vi "Inst.Transport.AppLauncher.vi"(8 "error in":errorcluster, 11 "Debug Mode":bool) -> (0 "error out":errorcluster)   [LabVIEW 2019, in "Inst.Transport.lvclass"]
uses:
  Inst.Transport.lvclass
  <vilib>/JKI/JKI SMO/SMO/Typedefs/SMOState --Enum.ctl
  <userlib>/LevyLab/Instrument Framework/Instrument/Instrument.lvclass
  <userlib>/LevyLab/Instrument Framework/Instrument UI/Instrument UI.lvclass
  C:/Program Files (x86)/National Instruments/LabVIEW 2019/vi.lib/JKI/JKI SMO/SMO/SMO.lvclass
  C:/Program Files (x86)/National Instruments/LabVIEW 2019/vi.lib/JKI/JKI SMO/SMO.UI/SMO.UI.lvclass
  C:/Program Files (x86)/National Instruments/LabVIEW 2019/user.lib/LevyLab/Instrument Framework/Instrument/Instrument.lvclass
  <vilib>/JKI/JKI SMO/SMO/SMO.lvclass/SMO.ctl
  <vilib>/JKI/JKI SMO/SMO/Private/ReftoDVR--SMO.vi
  <vilib>/JKI/JKI SMO/SMO/SMO.lvclass
  <vilib>/JKI/JKI SMO/SMO.UI/SMO.UI.lvclass
panel:
  in  "UI":bool
  in  "Examine Configuration.ini":bool
  in  "Splash Status":string="Push Start to Start..." caption="String"
  in  "Start Application":bool caption="Play"
  in  "Stop Application":bool caption="Stop"
  out "UI SMO State":T1=enum."Stopped"
  out "SMO State":T1
  # "Example Instrument SMO Test Launcher"
  # "For instructions on how to use the JKI State Machine Objects, examples and video tutorials, visit:\nhttp://jki.net/state-machine-objects/\n\nJKI State Machine Objects™\nhttp://jki.net/state-machine-objects/\nCopyright (C) 2005-2015, JKI <info@jki.net>\nALL RIGHTS RESERVED"
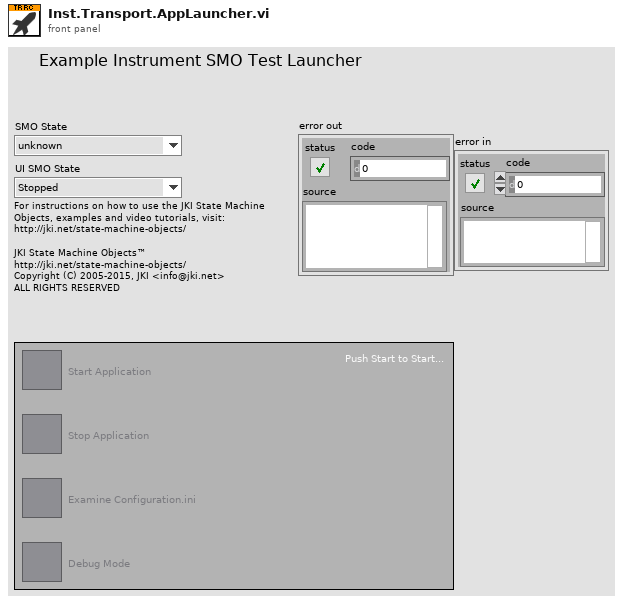
[diagram p1: front panel]
types:
  T1 = typedef "SMO.lvclass/SMOState --Enum.ctl" = enum16{"unknown", "Created", "Started", "Stopped"}
  T2 = enum32{"Invalid", "Standard", "Closed", "Hidden", "Minimized", "Maximized"}
  T3 = enum32{"invalid app kind", "Development System", "Run Time System", "Student Edition", "Embedded LabVIEW", "Evaluation", "Custom"}
  T4 = cluster{"Core":cluster{"Current VI Reference":refnum<vi>, "Close Panel on Exit?":bool}, "Instrument":refnum<class "Inst.Transport.lvclass">, "Instrument UI":refnum<class "Instrument UI.lvclass">}
  T5 = cluster{"Current VI Reference":refnum<vi>, "Close Panel on Exit?":bool}
  T6 = typedef "SMO.lvclass/Public Events.ctl" = cluster{"Error":refnum<user-event>, "State":refnum<user-event>, "Reserve State":refnum<user-event>}
  T7 = cluster{"Event Registration Refnum":refnum<event-registration>, "Event Registration Refnum":refnum<event-registration>}
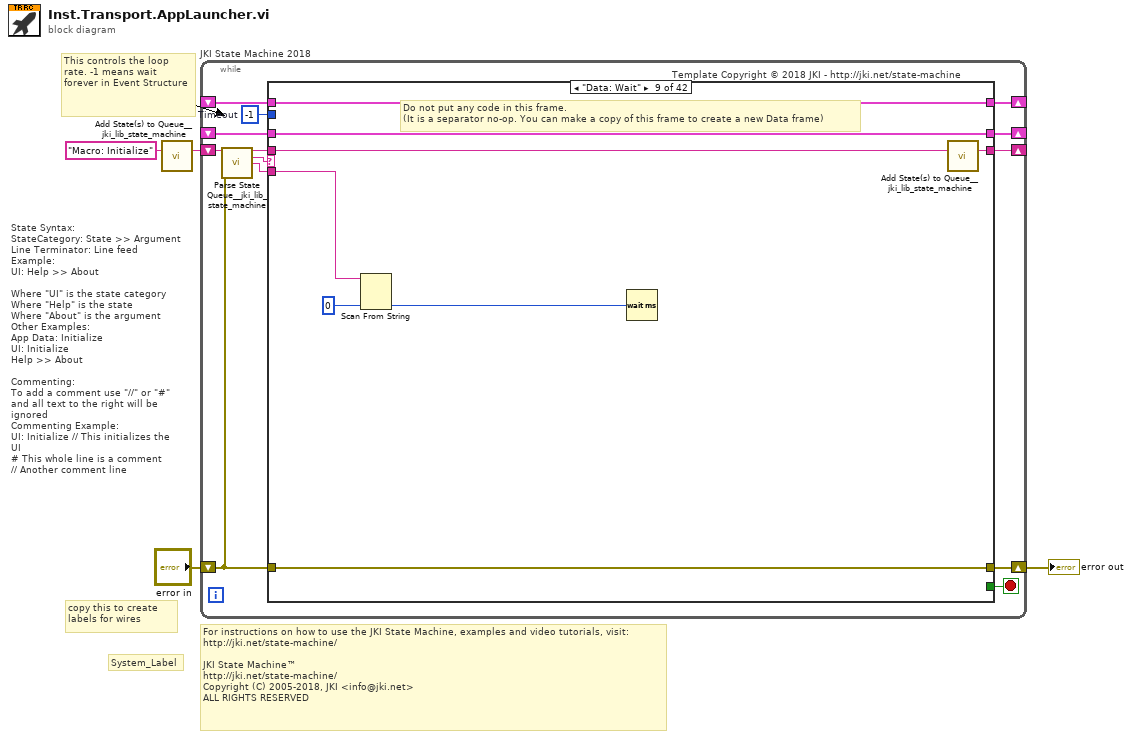
[diagram p0: block diagram]
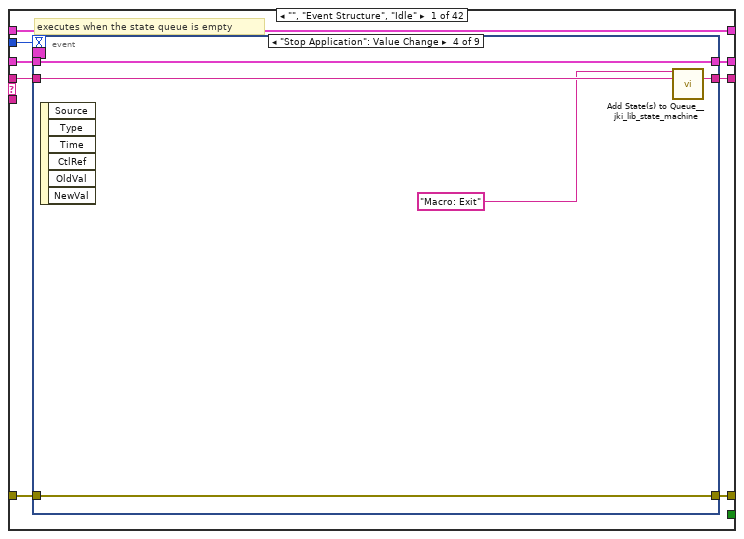
[diagram p2: hidden frame]
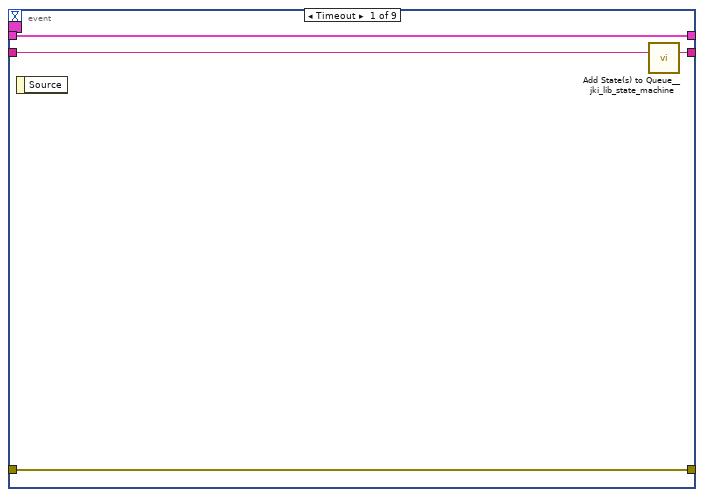
[diagram p3: hidden frame]
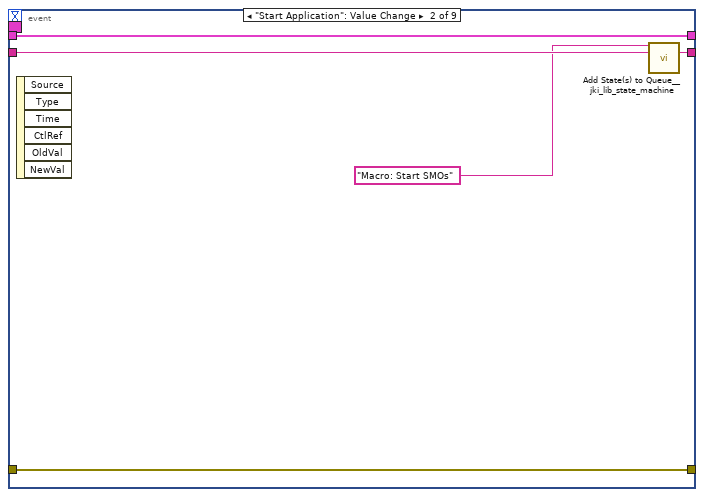
[diagram p4: hidden frame]
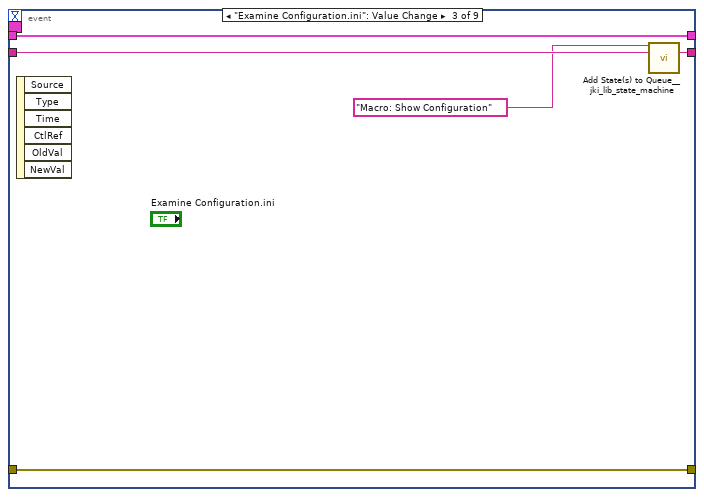
[diagram p5: hidden frame]
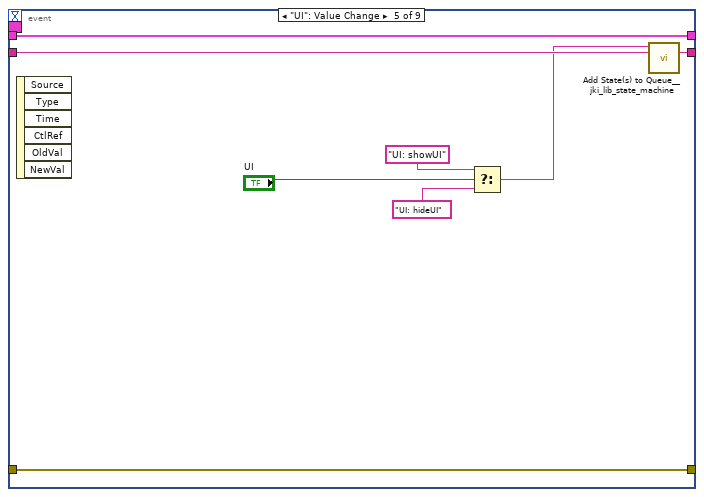
[diagram p6: hidden frame]
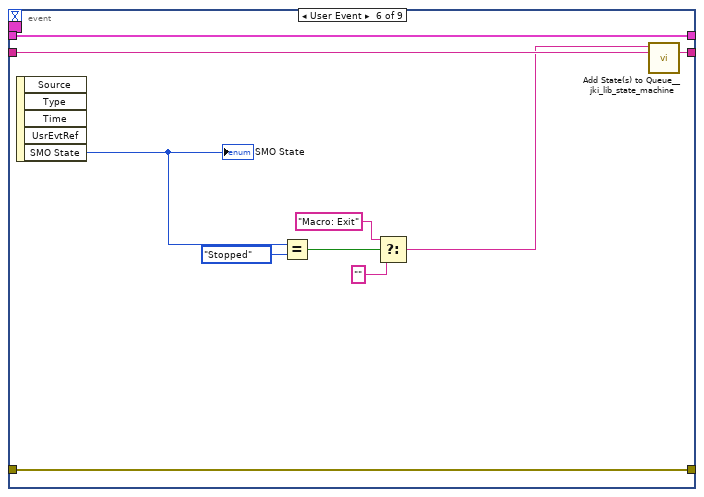
[diagram p7: hidden frame]
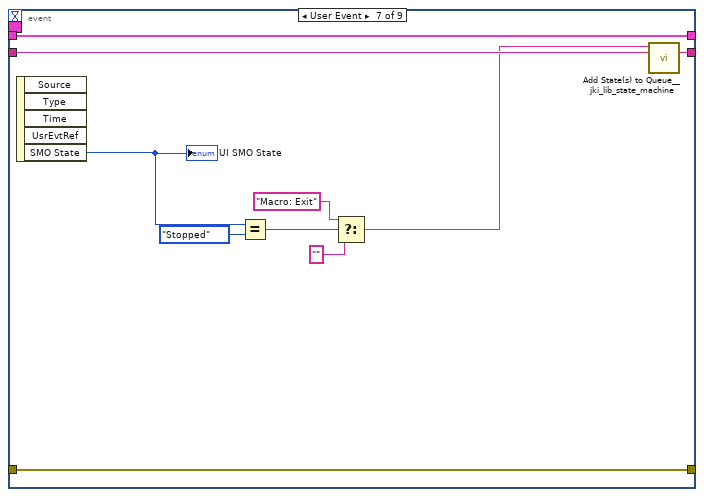
[diagram p8: hidden frame]
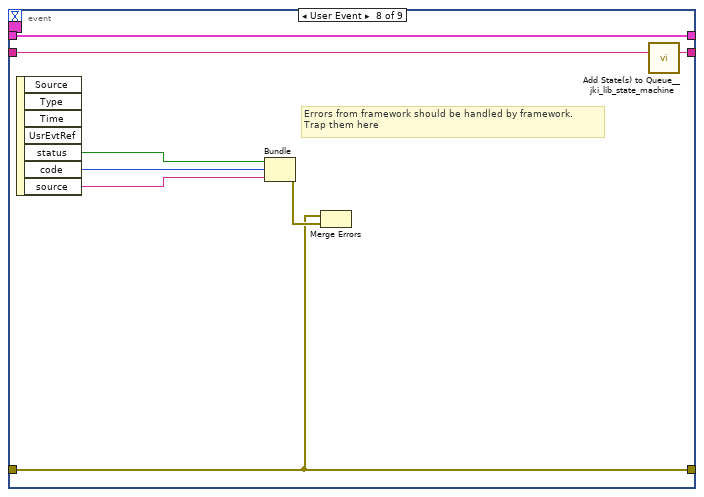
[diagram p9: hidden frame]
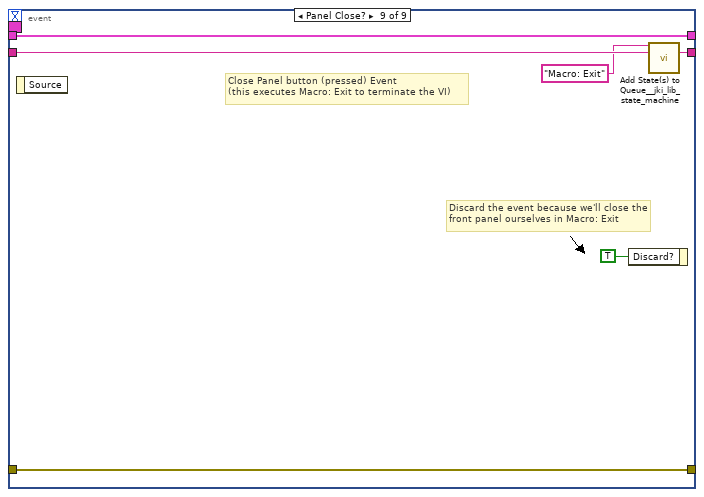
[diagram p10: hidden frame]
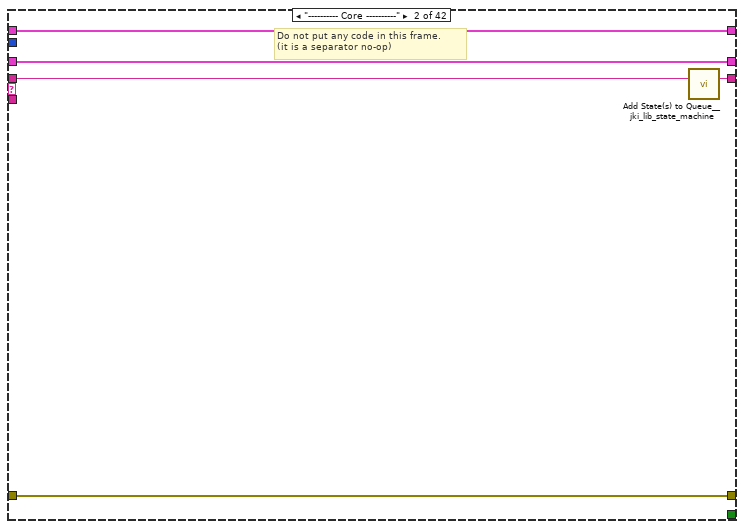
[diagram p11: hidden frame]
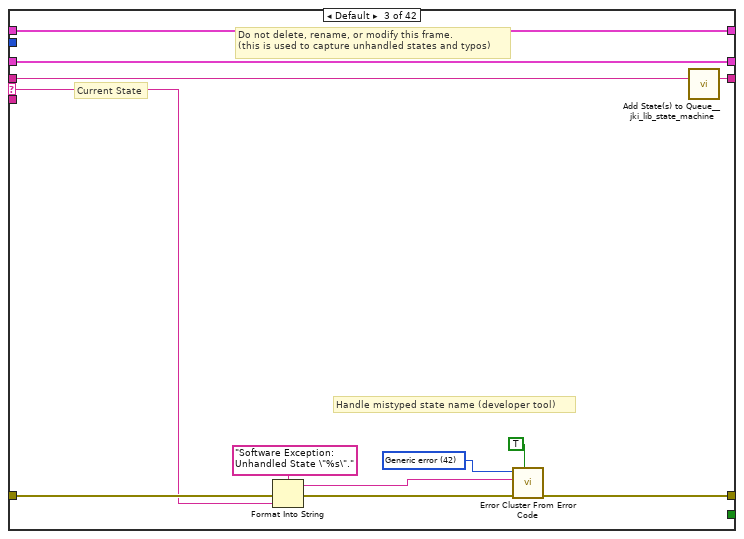
[diagram p12: hidden frame]
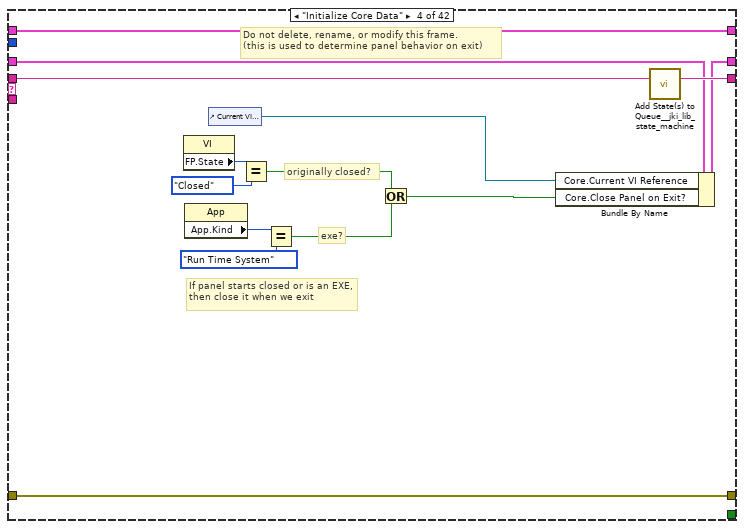
[diagram p13: hidden frame]
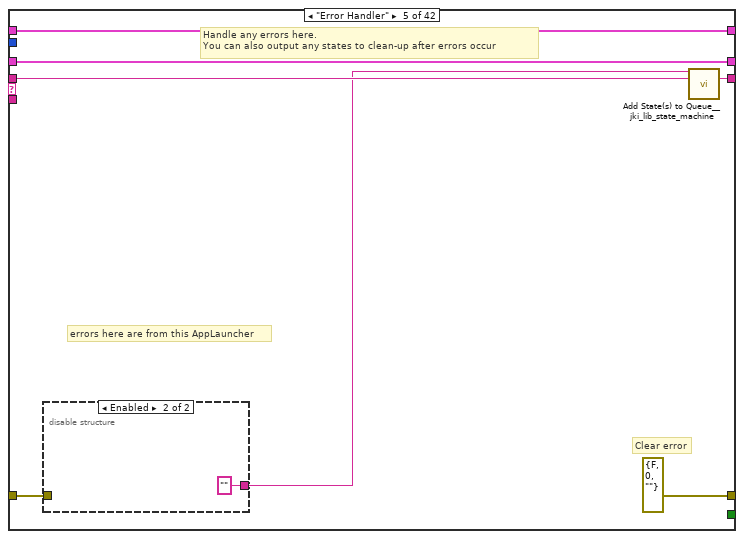
[diagram p14: hidden frame]
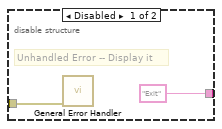
[diagram p15: hidden frame]
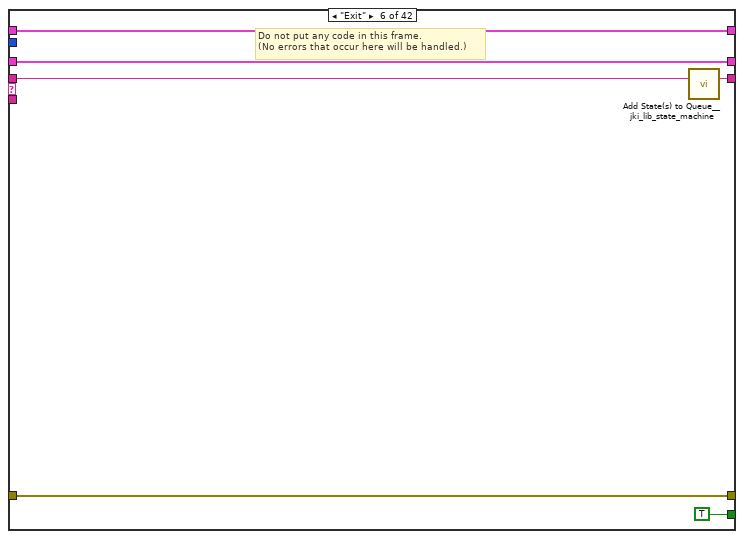
[diagram p16: hidden frame]
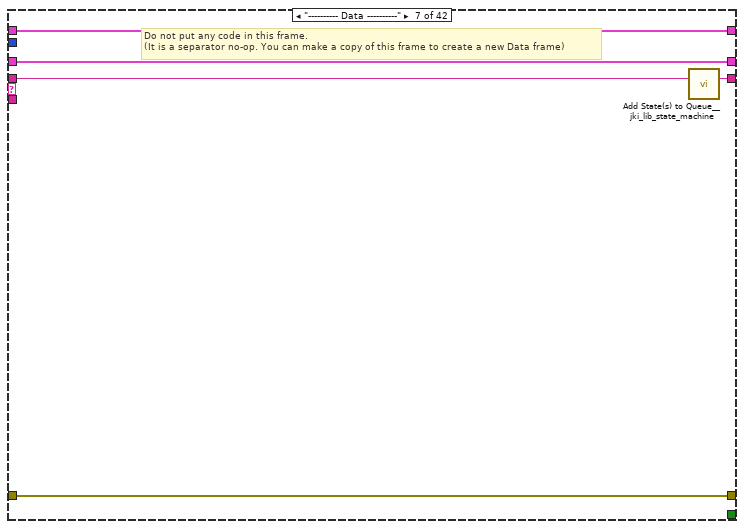
[diagram p17: hidden frame]
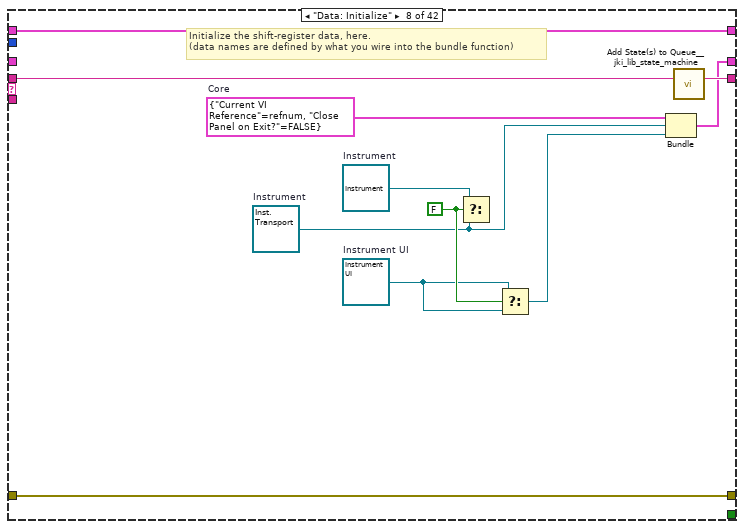
[diagram p18: hidden frame]
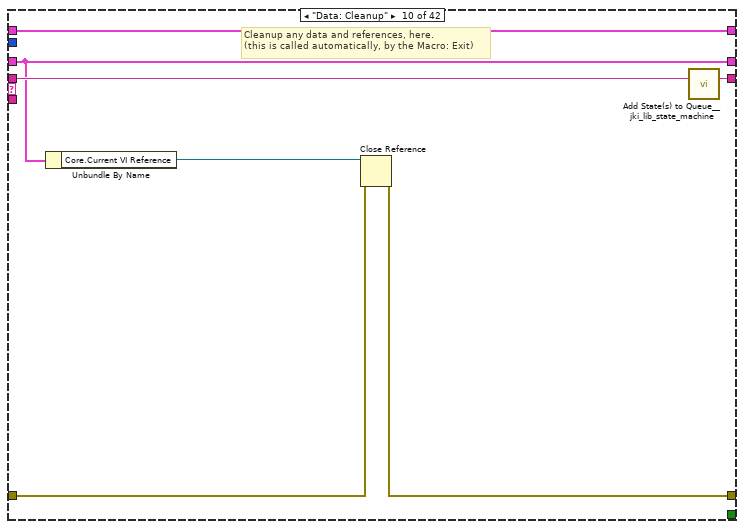
[diagram p19: hidden frame]
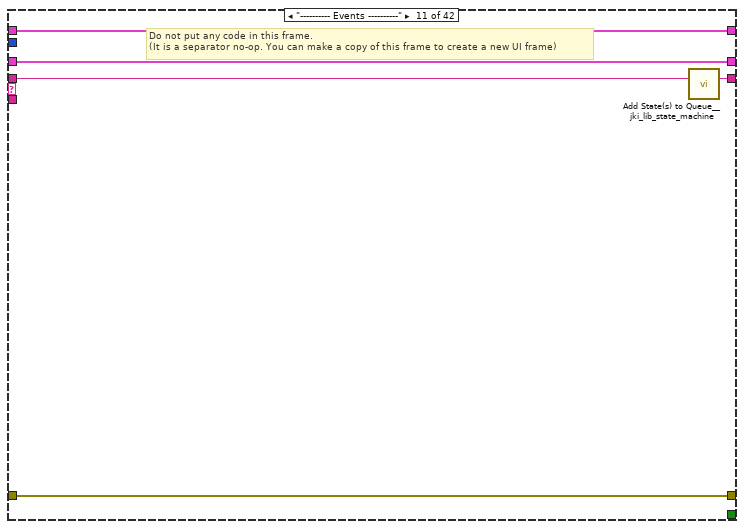
[diagram p20: hidden frame]
diagram:
  # "For instructions on how to use the JKI State Machine, examples and video tutorials, visit:\nhttp://jki.net/state-machine/\n\nJKI State Machine™\nhttp://jki.net/state-machine/\nCopyright (C) 2005-2018, JKI <info@jki.net>\nALL RIGHTS RESERVED"
  # "State Syntax:\nStateCategory: State >> Argument\nLine Terminator: Line feed\nExample:\nUI: Help >> About\n\nWhere \"UI\" is the state category\nWhere \"Help\" is the state\nWhere \"About\" is the argument\nOther Examples:\nApp Data: Initialize\nUI: Initialize\nHelp >> About\n\nCommenting:\nTo add a comment use \"//\" or \"#\" and all text to the right will be ignored\nCommenting Example:\nUI: Initialize // This initializes the UI\n# This whole line is a comment\n// Another comment line"
  # "copy this to create labels for wires"
  # "This controls the loop rate. -1 means wait forever in Event Structure"
  # "System_Label"
  n1 = call <vilib>:"Add State(s) to Queue__jki_lib_state_machine.vi"("State(s) in (\"\")"="Macro: Initialize") -> ("States Out"=w4:string)  [unwired: 14 in]
  n2 = while "JKI State Machine 2018" {
    shift-right: [w11] -> _
    shift-left: _ -> [w6]
    shift-right: [w14] -> w2
    shift-left: "error in" -> [w9]
    shift-right: [w13] -> _
    shift-left: w4 -> [w15]
    shift-right: [w8] -> _
    shift-left: _ -> [w7]
    stop <- w12 stop-if-true
    w10 = -1  # Timeout
    # "Template Copyright © 2018 JKI - http://jki.net/state-machine"
    n3 = call <vilib>:"Parse State Queue__jki_lib_state_machine.vi"("State Queue"=w15, "Error In (no error)"=w9) -> ("Remaining States"=w17:string, "Current State"=w5:string, "Arguments"=w16:string)  [unwired: 11 in]
    n4 = case shown="\"Data: Wait\"" w5 {
      selector: w5 -> [_ _ w93 _ _ _ _ _ _ _ _ _ _ _ _ _ _ _ _ _ _ _ _ _ _ _ _ _ _ _ _ _ _ _ _ _ _ _ _ _ _ _]
      tunnel: w17 -> [w25 w91 w97 w117 w124 w133 w138 w149 w157 w164 w169 w182 w193 w198 w206 w213 w225 w303 w310 w317 w324 w329 w334 w340 w346 w352 w358 w370 w375 w386 w397 w407 w414 w425 w440 w455 w470 w487 w502 w511 w518 w523]
      tunnel: w16 -> [_ _ _ _ _ _ _ _ w152 _ _ _ _ _ _ w208 w219 _ _ _ _ _ _ _ _ _ _ _ _ _ _ _ _ _ _ _ _ _ _ _ w515 _]
      tunnel: [w22 w89 w99 w114 errorcluster {"status"=FALSE, "code"=0, "source"=""} ("error out") w130 w136 w144 w155 w160 w167 w171 w188 w196 w201 w209 w222 w293 w307 w311 w318 w327 w332 w338 w344 w350 w356 w368 w373 w382 w389 w398 w408 w421 w436 w451 w467 w484 w499 w509 w513 w521] -> w14
      tunnel: w9 -> [w21 w89 w98 w114 w120 w130 w136 w144 w155 w161 w167 w173 w189 w196 w203 w210 w223 w294 w304 w312 w319 w327 w332 w338 w344 w350 w356 w368 w373 w383 w390 w399 w409 w418 w432 w448 w465 w482 w495 w509 w514 w521]
      tunnel: [w24 w90 w96 w116 w123 w132 w137 w148 w156 w163 w168 w181 w192 w197 w205 w212 w224 w302 w309 w316 w323 w328 w333 w339 w345 w351 w357 w369 w374 w385 w396 w406 w413 w424 w439 w454 w469 w486 w501 w510 w517 w522] -> w13
      tunnel: [_ _ _ _ _ TRUE _ _ _ _ _ _ _ _ _ _ _ _ _ _ _ _ _ _ _ _ _ _ _ _ _ _ _ _ _ _ _ _ _ _ _ _] -> w12
      tunnel: [w20 w88 w95 w115 w121 w131 w135 w147 w154 w159 w166 w176 w191 w195 w204 w211 w221 w291 w306 w314 w321 w326 w331 w337 w343 w349 w355 w367 w372 w381 w392 w403 w411 w422 w437 w452 w466 w483 w498 w508 w516 w520] -> w11
      tunnel: w10 -> [w19 _ _ _ _ _ _ _ _ _ _ _ _ _ _ _ _ _ _ _ _ _ _ _ _ _ _ _ _ _ _ _ _ _ _ _ _ _ _ _ _ _]
      tunnel: [w18 w87 w92 w104 w119 w128 w134 w145 w153 w158 w165 w179 w190 w194 w202 w207 w218 w292 w308 w315 w322 w325 w330 w335 w341 w348 w354 w361 w371 w384 w395 w405 w412 w423 w438 w453 w468 w485 w500 w507 w512 w519] -> w8
      tunnel: w7 -> [w18 w87 w92 w104 w119 w128 w134 w145 w153 w158 w165 _ w190 w194 w202 w207 w218 w292 w308 w315 w322 w325 w330 w335 w341 w348 w354 w361 w371 w384 w395 w405 w412 w423 w438 w453 w468 w485 w500 w507 w512 w519]
      tunnel: w6 -> [w23 w88 w95 w110 w121 w131 w135 _ w154 w159 w166 w176 w191 w195 w204 w211 w221 w291 w306 w314 w321 w326 w331 w337 w343 w349 w355 w367 w372 w379 w393 w404 w411 w422 w437 w452 w466 w483 w498 w508 w516 w520]
      frame "", "Event Structure", "Idle" {
        # "executes when the state queue is empty"
        n5 = event shown="[3] \"Stop Application\": Value Change" {
          selector: w18 -> [_ _ _ _ _ _ _ _ _]
          dyn-events: _ -> [_ _ _ _ _ _ _ _ _]
          timeout: w19 -> [_ _ _ _ _ _ _ _ _]
          tunnel: w25 -> [w29 w34 w39 w44 w52 w62 w72 w80 w86]
          tunnel: [w28 w33 w38 w43 w51 w61 w71 w79 w85] -> w24
          tunnel: w23 -> [w26 w31 w36 w41 w49 w59 w69 w78 w83]
          tunnel: [w27 w32 w37 w42 w50 w60 w70 w73 w84] -> w22
          tunnel: w21 -> [w27 w32 w37 w42 w50 w60 w70 w73 w84]
          tunnel: [w26 w31 w36 w41 w49 w59 w69 w78 w83] -> w20
          event Timeout {
            n6 = event-data() -> ()  [unwired: 1 in, 1 out]
            n7 = call <vilib>:"Add State(s) to Queue__jki_lib_state_machine.vi"("State(s) in (\"\")"=w29) -> ("States Out"=w28:string)  [unwired: 14 in]
          }
          event "Start Application": Value Change {
            n8 = event-data() -> ()  [unwired: 1 in, 6 out]
            n9 = call <vilib>:"Add State(s) to Queue__jki_lib_state_machine.vi"("State(s) in Front (\"\")"="Macro: Start SMOs" ("State(s) in Front (\"\")"), "State(s) in (\"\")"=w34) -> ("States Out"=w33:string)  [unwired: 13 in]
          }
          event "Examine Configuration.ini": Value Change {
            n10 = event-data() -> ()  [unwired: 1 in, 6 out]
            n11 = call <vilib>:"Add State(s) to Queue__jki_lib_state_machine.vi"("State(s) in Front (\"\")"="Macro: Show Configuration" ("State(s) in Front (\"\")"), "State(s) in (\"\")"=w39) -> ("States Out"=w38:string)  [unwired: 13 in]
          }
          event "Stop Application": Value Change {
            n12 = event-data() -> ()  [unwired: 1 in, 6 out]
            n13 = call <vilib>:"Add State(s) to Queue__jki_lib_state_machine.vi"("State(s) in Front (\"\")"="Macro: Exit" ("State(s) in Front (\"\")"), "State(s) in (\"\")"=w44) -> ("States Out"=w43:string)  [unwired: 13 in]
          }
          event "UI": Value Change {
            n14 = event-data() -> ()  [unwired: 1 in, 6 out]
            n15 = Select(t="UI: showUI" ("State(s) in Front (\"\")"), s="UI", f="UI: hideUI" ("State(s) in Front (\"\")")) -> (s? t:f=w46:string)
            n16 = call <vilib>:"Add State(s) to Queue__jki_lib_state_machine.vi"("State(s) in Front (\"\")"=w46, "State(s) in (\"\")"=w52) -> ("States Out"=w51:string)  [unwired: 13 in]
          }
          event User Event {
            n17 = event-data() -> ("SMO State"=w54:T1)  [unwired: 1 in, 4 out]
            "SMO State" <- w54
            n18 = Equal?(x=w54, y=SMOState_--Enum."Stopped") -> (x = y?=w57:bool)
            n19 = Select(t="Macro: Exit", s=w57, f="" ("State(s) in Front (\"\")")) -> (s? t:f=w53:string)
            n20 = call <vilib>:"Add State(s) to Queue__jki_lib_state_machine.vi"("State(s) in Front (\"\")"=w53, "State(s) in (\"\")"=w62) -> ("States Out"=w61:string)  [unwired: 13 in]
          }
          event User Event {
            n21 = event-data() -> ("SMO State"=w63:T1)  [unwired: 1 in, 4 out]
            "UI SMO State" <- w63
            n22 = Equal?(x=w63, y=SMOState_--Enum."Stopped") -> (x = y?=w67:bool)
            n23 = Select(t="Macro: Exit", s=w67, f="" ("State(s) in Front (\"\")")) -> (s? t:f=w65:string)
            n24 = call <vilib>:"Add State(s) to Queue__jki_lib_state_machine.vi"("State(s) in Front (\"\")"=w65, "State(s) in (\"\")"=w72) -> ("States Out"=w71:string)  [unwired: 13 in]
          }
          event User Event {
            # "Errors from framework should be handled by framework.\nTrap them here"
            n25 = event-data() -> ("status"=w74:bool, "code"=w76:i32, "source"=w75:string)  [unwired: 1 in, 4 out]
            n26 = Bundle("status"=w74, "code"=w76, "source"=w75) -> (w77:errorcluster)  [unwired: 1 in]
            n27 = Merge Errors(w73, w77) -> ()  [unwired: 1 out]
            n28 = call <vilib>:"Add State(s) to Queue__jki_lib_state_machine.vi"("State(s) in (\"\")"=w80) -> ("States Out"=w79:string)  [unwired: 14 in]
          }
          event Panel Close? {
            # "Discard the event because we'll close the front panel ourselves in Macro: Exit"
            # "Close Panel button (pressed) Event\n(this executes Macro: Exit to terminate the VI)"
            n29 = event-data() -> ()  [unwired: 1 in, 1 out]
            n30 = event-data("Discard?"=TRUE) -> ()  [unwired: 1 in, 1 out]
            n31 = call <vilib>:"Add State(s) to Queue__jki_lib_state_machine.vi"("State(s) in Front (\"\")"="Macro: Exit", "State(s) in (\"\")"=w86) -> ("States Out"=w85:string)  [unwired: 13 in]
          }
        }
      }
      frame "---------- Core ----------" {
        # "Do not put any code in this frame.\n(it is a separator no-op)"
        n32 = call <vilib>:"Add State(s) to Queue__jki_lib_state_machine.vi"("State(s) in (\"\")"=w91) -> ("States Out"=w90:string)  [unwired: 14 in]
      }
      frame Default {
        w102 = 42 items=["No error", "Argument error", "Memory is full", "Out of zone", "End of file", "File already open", "Generic file I/O error", "File not found", "File permission error", "Disk is full", "Duplicate path", "Too many files open", "System feature not enabled", "Resource file not found", "Cannot add resource", "Resource not found", "Image not found", "Image memory error", "Pen does not exist", "Config type invalid", "Config token not found", "Config parse error", "Config memory error", "Bad external code format", "Bad external code offset", "External code not present", "Null window", "Destroy window error", "Null menu", "Print aborted", "Bad print record", "Print driver error", "Windows error during printing", "Memory error during printing", "Print dialog error", "Generic print error", "Invalid device refnum", "Device not found", "Device parameter error", "Device unit error", "Cannot open device", "Device call aborted", "Generic error", "Cancelled by user", "Object ID too low", "Object ID too high", "Object not in heap", "Unknown heap", "Unknown object (invalid DefProc)", "Unknown object (DefProc not in table)", "Message out of range", "Invalid (null) method", "Unknown message", "Manager call not supported", "Bad address", "Network operation in progress", "Network operation timed out", "Connection is busy", "Network attribute not supported", "Network error", "Address in use", "System out of memory", "Connection aborted", "Connection refused", "Not connected", "Already connected", "Connection closed", "Initialization error (interapplication manager)", "Bad occurrence", "Wait on unbound occurrence handler", "Occurrence queue overflow", "Datalog type conflict", "Unused", "Unrecognized type (interapplication manager)", "Memory corrupt", "Failed to make temporary DLL", "Old CIN version", "Drag socket not found", "Failed to load drop-object", "Failed to register OLE object", "Failed to release OLE object", "Format specifier type mismatch", "Unknown format specifier", "Too few format specifiers", "Too many format specifiers", "Scan failed", "Newer CIN version", "Error converting to variant", "Runtime menu error", "Password tampered", "Variant attribute not found", "Incompatible variant data type", "Event data is not available", "Event Store is not present", "Occurrence is not found", "Event Queue is not created", "Event info is not available", "Refnum passed is NULL", "Error retrieving Class GUID", "Error retrieving CoClass GUID", "Error retrieving TypeLib GUID.", "Bad built application magic bytes.", "Specific driver is different from the specific driver associated with the Logical Name.", "There is no session opened to the class driver.", "Max Error", "MAX - Error with config objects", "MAX - Error loading configuration", "MAX - Group not supported"]
        # "Current State"
        # "Do not delete, rename, or modify this frame.\n(this is used to capture unhandled states and typos)"
        # "Handle mistyped state name (developer tool)"
        n33 = Format Into String(format string="Software Exception: Unhandled State \"%s\"." ("message"), error in=w98, w93) -> (resulting string=w101:string, error out=w100:errorcluster)  [unwired: 1 in]
        n34 = call <vilib>:"Error Cluster From Error Code.vi"("show call chain? (False)"=TRUE, "error in (no error)"=w100, "error message (\"\")"=w101, "error code (0)"=w102) -> ("error out"=w99:errorcluster)  [unwired: 5 in]
        n35 = call <vilib>:"Add State(s) to Queue__jki_lib_state_machine.vi"("State(s) in (\"\")"=w97) -> ("States Out"=w96:string)  [unwired: 14 in]
      }
      frame "Initialize Core Data" {
        # "Do not delete, rename, or modify this frame.\n(this is used to determine panel behavior on exit)"
        # "originally closed?"
        # "exe?"
        # "If panel starts closed or is an EXE, then close it when we exit"
        n36 = property class="VI"() -> ("FP.State"=w107:T2)  [unwired: 2 in, 2 out]
        n37 = property class="App"() -> ("App.Kind"=w113:T3)  [unwired: 2 in, 2 out]
        n38 = control-ref of="Current VI Reference"() -> (w108:refnum<vi>)
        n39 = Equal?(x=w107, y=T2."Closed" ("Front Panel Window:State")) -> (x = y?=w105:bool)
        n40 = Equal?(x=w113, y=T3."Run Time System" ("Application:Kind")) -> (x = y?=w111:bool)
        n41 = Or(x=w105, y=w111) -> (x .or. y?=w109:bool)
        n42 = Bundle By Name(cluster=w110, "Core.Current VI Reference"=w108, "Core.Close Panel on Exit?"=w109) -> (w115:T4)
        n43 = call <vilib>:"Add State(s) to Queue__jki_lib_state_machine.vi"("State(s) in (\"\")"=w117) -> ("States Out"=w116:string)  [unwired: 14 in]
      }
      frame "Error Handler" {
        # "errors here are from this AppLauncher"
        # "Handle any errors here.\nYou can also output any states to clean-up after errors occur"
        # "Clear error"
        n44 = disable-structure shown="Enabled" {
          disable-tunnel: w120 -> [w126 _]
          disable-tunnel: ["Exit" "" ("State(s) in Front (\"\")")] -> w118
          frame Disabled {
            # "Unhandled Error -- Display it"
            n45 = call <vilib>:"General Error Handler.vi"("error in (no error)"=w126) -> ()  [unwired: 10 in, 5 out]
          }
          frame Enabled {
          }
        }
        n46 = call <vilib>:"Add State(s) to Queue__jki_lib_state_machine.vi"("State(s) in Front (\"\")"=w118, "State(s) in (\"\")"=w124) -> ("States Out"=w123:string)  [unwired: 13 in]
      }
      frame "Exit" {
        # "Do not put any code in this frame.\n(No errors that occur here will be handled.)"
        n47 = call <vilib>:"Add State(s) to Queue__jki_lib_state_machine.vi"("State(s) in (\"\")"=w133) -> ("States Out"=w132:string)  [unwired: 14 in]
      }
      frame "---------- Data ----------" {
        # "Do not put any code in this frame.\n(It is a separator no-op. You can make a copy of this frame to create a new Data frame)"
        n48 = call <vilib>:"Add State(s) to Queue__jki_lib_state_machine.vi"("State(s) in (\"\")"=w138) -> ("States Out"=w137:string)  [unwired: 14 in]
      }
      frame "Data: Initialize" {
        w142 = FALSE ("s")
        w141 = refnum<class "Inst.Transport.lvclass"> refnum  # Instrument
        w140 = refnum<class "Instrument UI.lvclass"> refnum  # Instrument UI
        w143 = refnum<class "Instrument.lvclass"> refnum  # Instrument
        w146 = T5 {"Current VI Reference"=refnum, "Close Panel on Exit?"=FALSE}  # Core
        # "Initialize the shift-register data, here.\n(data names are defined by what you wire into the bundle function)"
        n49 = Select(t=w143, s=w142, f=w141) -> ()  [unwired: 1 out]
        n50 = Select(t=w140, s=w142, f=w140) -> (s? t:f=w139:refnum<class "Instrument UI.lvclass">)
        n51 = Bundle("Core"=w146, "Instrument"=w141, "Instrument UI"=w139) -> (w147:T4)  [unwired: 1 in]
        n52 = call <vilib>:"Add State(s) to Queue__jki_lib_state_machine.vi"("State(s) in (\"\")"=w149) -> ("States Out"=w148:string)  [unwired: 14 in]
      }
      frame "Data: Wait" {
        # "Do not put any code in this frame.\n(It is a separator no-op. You can make a copy of this frame to create a new Data frame)"
        n53 = Scan From String(input string=w152, default 1=u32 0) -> (output 1=w150:u32)  [unwired: 3 in, 3 out]
        n54 = Wait (ms)(milliseconds to wait=w150) -> ()  [unwired: 1 out]
        n55 = call <vilib>:"Add State(s) to Queue__jki_lib_state_machine.vi"("State(s) in (\"\")"=w157) -> ("States Out"=w156:string)  [unwired: 14 in]
      }
      frame "Data: Cleanup" {
        # "Cleanup any data and references, here.\n(this is called automatically, by the Macro: Exit)"
        n56 = Unbundle By Name(w159) -> ("Core.Current VI Reference"=w162:refnum<vi>)
        n57 = Close Reference(reference=w162, error in (no error)=w161) -> (error out=w160:errorcluster)
        n58 = call <vilib>:"Add State(s) to Queue__jki_lib_state_machine.vi"("State(s) in (\"\")"=w164) -> ("States Out"=w163:string)  [unwired: 14 in]
      }
      frame "---------- Events ----------" {
        # "Do not put any code in this frame.\n(It is a separator no-op. You can make a copy of this frame to create a new UI frame)"
        n59 = call <vilib>:"Add State(s) to Queue__jki_lib_state_machine.vi"("State(s) in (\"\")"=w169) -> ("States Out"=w168:string)  [unwired: 14 in]
      }
      frame "Events: Register" {
        # "Do not put any code in this frame.\n(It is a separator no-op. You can make a copy of this frame to create a new UI frame)"
        n60 = Unbundle By Name(w176) -> ("Instrument"=w175:refnum<class "Inst.Transport.lvclass">, "Instrument UI"=w174:refnum<class "Instrument UI.lvclass">)
        n61 = call <vilib>:"GetPublicEvents.vi"("error in (no error)"=w173, "SMO"=w175) -> ("error out"=w172:errorcluster, "Public Events"=w177:T6)  [unwired: 7 in, 1 out]
        n62 = disable-structure shown="Enabled" {
          disable-tunnel: [w186 _] -> w178
          disable-tunnel: w174 -> [w185 _]
          disable-tunnel: w172 -> [w184 w187]
          disable-tunnel: [w183 w187] -> w171
          frame Disabled {
            n63 = call <vilib>:"GetPublicEvents.vi"("error in (no error)"=w184, "SMO"=w185) -> ("error out"=w183:errorcluster, "Public Events"=w186:T6)  [unwired: 7 in, 1 out]
          }
          frame Enabled {
          }
        }
        n64 = register-events(w177) -> (reference out=w180:refnum<event-registration>)  [unwired: 2 in, 1 out]
        n65 = register-events(w178) -> (reference out=w170:refnum<event-registration>)  [unwired: 2 in, 1 out]
        n66 = Bundle("Event Registration Refnum"=w180, "Event Registration Refnum"=w170) -> (w179:T7)  [unwired: 1 in]
        n67 = call <vilib>:"Add State(s) to Queue__jki_lib_state_machine.vi"("State(s) in (\"\")"=w182) -> ("States Out"=w181:string)  [unwired: 14 in]
      }
      frame "Events: Unregister" {
        # "Do not put any code in this frame.\n(It is a separator no-op. You can make a copy of this frame to create a new UI frame)"
        n68 = Unregister For Events(event registration refnum=w190, error in=w189) -> (error out=w188:errorcluster)
        n69 = call <vilib>:"Add State(s) to Queue__jki_lib_state_machine.vi"("State(s) in (\"\")"=w193) -> ("States Out"=w192:string)  [unwired: 14 in]
      }
      frame "---------- UI ----------" {
        # "Do not put any code in this frame.\n(It is a separator no-op. You can make a copy of this frame to create a new UI frame)"
        n70 = call <vilib>:"Add State(s) to Queue__jki_lib_state_machine.vi"("State(s) in (\"\")"=w198) -> ("States Out"=w197:string)  [unwired: 14 in]
      }
      frame "UI: Initialize" {
        # "Initialize the User Interface, here.\n(this is called automatically, by the Macro: Init)"
        n71 = invoke on="Stop Application" class="Bool" method="Reinit To Default"() -> ()  [unwired: 3 in, 3 out]
        n72 = invoke on="error out" class="Clust (strict)" method="Reinit To Default"() -> ()  [unwired: 3 in, 3 out]
        n73 = invoke on="SMO State" class="Enum (strict)" method="Reinit To Default"() -> ()  [unwired: 3 in, 3 out]
        n74 = invoke on="Start Application" class="Bool" method="Reinit To Default"() -> ()  [unwired: 3 in, 3 out]
        n75 = call <userlib>:"Fit VI window to Largest Dec__ogtk.vi"("error in (no error)"=w203, "border spacing (2 px)"=1) -> ("error out"=w201:errorcluster)  [unwired: 4 in, 1 out]
        n76 = property on="UI" class="Bool (strict)"("Visible"=FALSE) -> ()  [unwired: 2 in, 2 out]
        n77 = call <vilib>:"Add State(s) to Queue__jki_lib_state_machine.vi"("State(s) in (\"\")"=w206) -> ("States Out"=w205:string)  [unwired: 14 in]
      }
      frame "UI: Cursor Set" {
        # "Argument"
        # "Set and Unset Cursor Busy.\n(Usage: \"UI: Cursor Set >> Busy|Idle\")"
        n78 = case shown="\"Busy\"" w208 {
          tunnel: w210 -> [w215 w217]
          tunnel: [w214 w216] -> w209
          frame "Idle", Default {
            n79 = call <vilib>:"Unset Busy.vi"("error in (no error)"=w215) -> ("error out"=w214:errorcluster)  [unwired: 10 in]
          }
          frame "Busy" {
            n80 = call <vilib>:"Set Busy.vi"("error in (no error)"=w217) -> ("error out"=w216:errorcluster)  [unwired: 9 in, 1 out]
          }
        }
        n81 = call <vilib>:"Add State(s) to Queue__jki_lib_state_machine.vi"("State(s) in (\"\")"=w213) -> ("States Out"=w212:string)  [unwired: 14 in]
      }
      frame "UI: Front Panel State" {
        # "Argument"
        # "Set Front Panel Open or Closed\n(Usage: \"UI: Front Panel State >> Open|Close\")"
        n82 = Unbundle By Name(w221) -> ("Core.Current VI Reference"=w220:refnum<vi>)
        n83 = case shown="\"Open\", \"Standard\", Default" w219 {
          tunnel: w223 -> [w231 w246 w257 w270 w283]
          tunnel: [w233 w247 w259 w272 w285] -> w222
          tunnel: w220 -> [w232 w244 w258 w271 w284]
          frame "Open", "Standard", Default {
            w226 = T2."Standard" ("State")
            n84 = property class="VI"(reference=w232, error in=w231) -> (reference out=w229:refnum<vi>, error out=w230:errorcluster, "FP.State"=w228:T2)
            n85 = Not Equal?(x=w228, y=w226) -> (x != y?=w227:bool)
            n86 = case shown="False" w227 {
              tunnel: [w237 w239] -> w233
              tunnel: w230 -> [w236 w239]
              tunnel: w229 -> [w235 _]
              tunnel: w226 -> [w234 _]
              frame True {
                n87 = invoke class="VI" method="FP.Open"(reference=w235, error in=w236, "Activate"=TRUE, "State"=w234) -> (error out=w237:errorcluster)  [unwired: 1 in, 4 out]
              }
              frame False {
              }
            }
          }
          frame "Close", "Closed" {
            n88 = property class="VI"(reference=w244, error in=w246) -> (reference out=w243:refnum<vi>, error out=w245:errorcluster, "FP.State"=w241:T2)
            n89 = Not Equal?(x=w241, y=T2."Closed" ("Front Panel Window:State")) -> (x != y?=w240:bool)
            n90 = case shown="True" w240 {
              tunnel: [w248 w251] -> w247
              tunnel: w245 -> [w248 w250]
              tunnel: w243 -> [_ w249]
              frame False {
              }
              frame True {
                n91 = invoke class="VI" method="FP.Close"(reference=w249, error in=w250) -> (error out=w251:errorcluster)  [unwired: 1 in, 2 out]
              }
            }
          }
          frame "Hidden", "Hide" {
            w252 = T2."Hidden" ("State")
            n92 = property class="VI"(reference=w258, error in=w257) -> (reference out=w255:refnum<vi>, error out=w256:errorcluster, "FP.State"=w254:T2)
            n93 = Not Equal?(x=w254, y=w252) -> (x != y?=w253:bool)
            n94 = case shown="True" w253 {
              tunnel: [w263 w264] -> w259
              tunnel: w256 -> [w262 w264]
              tunnel: w255 -> [w261 _]
              tunnel: w252 -> [w260 _]
              frame True {
                n95 = invoke class="VI" method="FP.Open"(reference=w261, error in=w262, "State"=w260) -> (error out=w263:errorcluster)  [unwired: 2 in, 4 out]
              }
              frame False {
              }
            }
          }
          frame "Minimize", "Minimized" {
            w265 = T2."Minimized" ("State")
            n96 = property class="VI"(reference=w271, error in=w270) -> (reference out=w268:refnum<vi>, error out=w269:errorcluster, "FP.State"=w267:T2)
            n97 = Not Equal?(x=w267, y=w265) -> (x != y?=w266:bool)
            n98 = case shown="True" w266 {
              tunnel: [w276 w277] -> w272
              tunnel: w269 -> [w275 w277]
              tunnel: w268 -> [w274 _]
              tunnel: w265 -> [w273 _]
              frame True {
                n99 = invoke class="VI" method="FP.Open"(reference=w274, error in=w275, "State"=w273) -> (error out=w276:errorcluster)  [unwired: 2 in, 4 out]
              }
              frame False {
              }
            }
          }
          frame "Maximize", "Maximized" {
            w278 = T2."Maximized" ("State")
            n100 = property class="VI"(reference=w284, error in=w283) -> (reference out=w281:refnum<vi>, error out=w282:errorcluster, "FP.State"=w280:T2)
            n101 = Not Equal?(x=w280, y=w278) -> (x != y?=w279:bool)
            n102 = case shown="True" w279 {
              tunnel: [w289 w290] -> w285
              tunnel: w282 -> [w288 w290]
              tunnel: w281 -> [w287 _]
              tunnel: w278 -> [w286 _]
              frame True {
                n103 = invoke class="VI" method="FP.Open"(reference=w287, error in=w288, "State"=w286) -> (error out=w289:errorcluster)  [unwired: 2 in, 4 out]
              }
              frame False {
              }
            }
          }
        }
        n104 = call <vilib>:"Add State(s) to Queue__jki_lib_state_machine.vi"("State(s) in (\"\")"=w225) -> ("States Out"=w224:string)  [unwired: 14 in]
      }
      frame "UI: Set Background Color" {
        # "Do not put any code in this frame.\n(It is a separator no-op. You can make a copy of this frame to create a new UI frame)"
        n105 = property class="VI"(error in=w294) -> (error out=w296:errorcluster, "Panel"=w297:refnum<vi>)  [unwired: 1 in, 1 out]
        n106 = property class="Pnl"(reference=w297, error in=w296) -> (error out=w295:errorcluster, "Panes[]"=w298:refnum<vi>[])  [unwired: 1 out]
        n107 = Index Array(array=w298, index=0) -> (element=w300:refnum<vi>)
        n108 = property class="Pane"(reference=w300, error in=w295, "PaneColor"=u32 16777238 ("Color Box")) -> (error out=w293:errorcluster)  [unwired: 1 out]
        n109 = call <vilib>:"Add State(s) to Queue__jki_lib_state_machine.vi"("State(s) in (\"\")"=w303) -> ("States Out"=w302:string)  [unwired: 14 in]
      }
      frame "UI: Open Configuration.ini" {
        # "Do not put any code in this frame.\n(It is a separator no-op. You can make a copy of this frame to create a new UI frame)"
        n110 = Unbundle By Name(w306) -> ("Instrument"=w305:refnum<class "Inst.Transport.lvclass">)
        n111 = call <userlib>:"Examine Configuration.vi"("error in (no error)"=w304, "Instrument in"=w305) -> ("error out"=w307:errorcluster)  [unwired: 8 in, 1 out]
        n112 = call <vilib>:"Add State(s) to Queue__jki_lib_state_machine.vi"("State(s) in (\"\")"=w310) -> ("States Out"=w309:string)  [unwired: 14 in]
      }
      frame "UI: showUI" {
        # "Do not put any code in this frame.\n(It is a separator no-op. You can make a copy of this frame to create a new UI frame)"
        n113 = Unbundle By Name(w314) -> ("Instrument"=w313:refnum<class "Inst.Transport.lvclass">)
        n114 = call "showUI.vi"("error in (no error)"=w312, "Inst.Transport in"=w313) -> ("error out"=w311:errorcluster)  [unwired: 8 in, 1 out]
        n115 = call <vilib>:"Add State(s) to Queue__jki_lib_state_machine.vi"("State(s) in (\"\")"=w317) -> ("States Out"=w316:string)  [unwired: 14 in]
      }
      frame "UI: hideUI" {
        # "Do not put any code in this frame.\n(It is a separator no-op. You can make a copy of this frame to create a new UI frame)"
        n116 = Unbundle By Name(w321) -> ("Instrument"=w320:refnum<class "Inst.Transport.lvclass">)
        n117 = call "hideUI.vi"("error in (no error)"=w319, "Inst.Transport in"=w320) -> ("error out"=w318:errorcluster)  [unwired: 8 in, 1 out]
        n118 = call <vilib>:"Add State(s) to Queue__jki_lib_state_machine.vi"("State(s) in (\"\")"=w324) -> ("States Out"=w323:string)  [unwired: 14 in]
      }
      frame "UI: Exit" {
        # "Do not put any code in this frame.\n(It is a separator no-op. You can make a copy of this frame to create a new UI frame)"
        n119 = invoke on="Start Application" class="Bool" method="Reinit To Default"() -> ()  [unwired: 3 in, 3 out]
        n120 = invoke on="Stop Application" class="Bool" method="Reinit To Default"() -> ()  [unwired: 3 in, 3 out]
        n121 = call <vilib>:"Add State(s) to Queue__jki_lib_state_machine.vi"("State(s) in (\"\")"=w329) -> ("States Out"=w328:string)  [unwired: 14 in]
      }
      frame "---------- Macro ----------" {
        # "Do not put any code in this frame.\n(It is a separator no-op. You can make a copy of this frame to create a new Macro frame)"
        n122 = call <vilib>:"Add State(s) to Queue__jki_lib_state_machine.vi"("State(s) in (\"\")"=w334) -> ("States Out"=w333:string)  [unwired: 14 in]
      }
      frame "Macro: Initialize" {
        # "Initialization Macro\n(This is called once, when the VI starts)"
        n123 = call <vilib>:"Add State(s) to Queue__jki_lib_state_machine.vi"("State(s) in Front (\"\")"="Data: Initialize\nInitialize Core Data\n//Events: Register\nUI: Initialize\nUI: Front Panel State >> Open\nUI: Set Background Color\nSplash: Set Status >> ...", "State(s) in (\"\")"=w340) -> ("States Out"=w339:string)  [unwired: 13 in]
      }
      frame "Macro: Show Configuration" {
        # "Initialization Macro\n(This is called once, when the VI starts)"
        n124 = call <vilib>:"Add State(s) to Queue__jki_lib_state_machine.vi"("State(s) in Front (\"\")"="Splash: Set Status >> Opeing Configuration...\nUI: Open Configuration.ini\nData: Wait >> 1000\nSplash: Set Status >> ...", "State(s) in (\"\")"=w346) -> ("States Out"=w345:string)  [unwired: 13 in]
      }
      frame "Macro: Start SMOs" {
        # "Do not put any code in this frame.\n(It is a separator no-op. You can make a copy of this frame to create a new Macro frame)"
        n125 = call <vilib>:"Add State(s) to Queue__jki_lib_state_machine.vi"("State(s) in Front (\"\")"="Splash: Set Status >> Creating Instrument...\nSMO: Create Instrument\nData: Wait >> 100\n//Splash: Set Status >> Creating Instrument UI...\n//SMO: Create Instrument UI\n//Data: Wait >> 100\nSplash: Set Status >> Registering Events...\nEvents: Register\nData: Wait >> 100\nSplash: Set Status >> Starting Instrument...\nSMO: Start Instrument\nData: Wait >> 100\nSplash: Set Status >> Instrument Process Started...\nData: Wait >> 100\n//Splash: Set Status >> Starting User Interface...\n//SMO: Start Instrument UI\n//Data: Wait >> 100\nUI: Front Panel State >> Hide\nSMO: Show Instrument UI" ("State(s) in Front (\"\")"), "State(s) in (\"\")"=w352) -> ("States Out"=w351:string)  [unwired: 13 in]
      }
      frame "Macro: Stop SMOs" {
        # "#todo\nshould stopping UI go before stopping Instrument?"
        # "Do not put any code in this frame.\n(It is a separator no-op. You can make a copy of this frame to create a new Macro frame)"
        n126 = call <vilib>:"Add State(s) to Queue__jki_lib_state_machine.vi"("State(s) in Front (\"\")"="UI: Front Panel State >> Show\nSplash: Set Status >> Stopping Instrument...\nSMO: Stop Instrument\nData: Wait >> 100\nSplash: Set Status >> Destroying Instrument...\nSMO: Destroy Instrument\nData: Wait >> 100\n//Splash: Set Status >>Hiding UI...\n//SMO: Hide Instrument UI\n//Data: Wait >> 100\n//Splash: Set Status >> Stopping UI...\n//SMO: Stop Instrument UI\n//Data: Wait >> 100\n//Splash: Set Status >> Destroying UI...\n//SMO: Destroy Instrument UI" ("State(s) in Front (\"\")"), "State(s) in (\"\")"=w358) -> ("States Out"=w357:string)  [unwired: 13 in]
      }
      frame "Macro: Exit" {
        # "Exit Macro\n(This is called once, when the VI exits)"
        n127 = Unbundle By Name(w367) -> ("Core.Close Panel on Exit?"=w366:bool)
        n128 = Select(t="UI: Front Panel State >> Close", s=w366, f="" ("Empty String Constant")) -> (s? t:f=w363:string)
        n129 = call <vilib>:"Add State(s) to Queue__jki_lib_state_machine.vi"("State(s) in Front (\"\")"="UI: Front Panel State >> Open\nUI: Exit\nMacro: Stop SMOs", "State(s) in (\"\")"=w363, "State(s) at Back (\"\")"="Data: Cleanup\nEvents: Unregister\nExit") -> ("States Out"=w362:string)  [unwired: 12 in]
        n130 = call <vilib>:"Add State(s) to Queue__jki_lib_state_machine.vi"("State(s) in Front (\"\")"=w362, "State(s) in (\"\")"=w370) -> ("States Out"=w369:string)  [unwired: 13 in]
      }
      frame "---------- SMO ----------" {
        # "Do not put any code in this frame.\n(It is a separator no-op. You can make a copy of this frame to create a new Macro frame)"
        n131 = call <vilib>:"Add State(s) to Queue__jki_lib_state_machine.vi"("State(s) in (\"\")"=w375) -> ("States Out"=w374:string)  [unwired: 14 in]
      }
      frame "SMO: Create Instrument" {
        # "Do not put any code in this frame.\n(It is a separator no-op. You can make a copy of this frame to create a new Macro frame)"
        n132 = Unbundle By Name(w379) -> ("Instrument"=w378:refnum<class "Inst.Transport.lvclass">)
        n133 = call <userlib>:"Create Instrument SMO.vi"("error in (no error)"=w383, "Debug Mode? [F]"="Debug Mode", "Configuration Window? [T]"=FALSE ("Config Window"), "Instrument in"=w378) -> ("error out"=w382:errorcluster, "Instrument out"=w380:refnum<class "Inst.Transport.lvclass">)  [unwired: 6 in]
        n134 = Bundle By Name(cluster=w379, "Instrument"=w380) -> (w381:T4)
        n135 = call <vilib>:"Add State(s) to Queue__jki_lib_state_machine.vi"("State(s) in (\"\")"=w386) -> ("States Out"=w385:string)  [unwired: 14 in]
      }
      frame "SMO: Start Instrument" {
        # "Do not put any code in this frame.\n(It is a separator no-op. You can make a copy of this frame to create a new Macro frame)"
        n136 = Unbundle By Name(w393) -> ("Instrument"=w394:refnum<class "Inst.Transport.lvclass">)
        n137 = call <vilib>:"Start.vi"("error in (no error)"=w390, "SMO"=w394) -> ("error out"=w389:errorcluster, "SMO out"=w391:refnum<class "Inst.Transport.lvclass">)  [unwired: 8 in]
        n138 = Bundle By Name(cluster=w393, "Instrument"=w391) -> (w392:T4)
        n139 = local write "UI"(TRUE ("UI")) -> ()
        n140 = property on="UI" class="Bool (strict)"("Visible"=TRUE) -> ()  [unwired: 2 in, 2 out]
        n141 = call <vilib>:"Add State(s) to Queue__jki_lib_state_machine.vi"("State(s) in (\"\")"=w397) -> ("States Out"=w396:string)  [unwired: 14 in]
      }
      frame "SMO: Create Instrument UI" {
        # "Do not put any code in this frame.\n(It is a separator no-op. You can make a copy of this frame to create a new Macro frame)"
        n142 = Unbundle By Name(w404) -> ("Instrument UI"=w402:refnum<class "Instrument UI.lvclass">, "Instrument"=w401:refnum<class "Inst.Transport.lvclass">)
        n143 = call <userlib>:"Create UI.vi"("error in (no error)"=w399, "Instrument in"=w401, "Instrument UI"=w402) -> ("error out"=w398:errorcluster, "Instrument UI out"=w400:refnum<class "Instrument UI.lvclass">)  [unwired: 7 in]
        n144 = Bundle By Name(cluster=w404, "Instrument UI"=w400) -> (w403:T4)
        n145 = call <vilib>:"Add State(s) to Queue__jki_lib_state_machine.vi"("State(s) in (\"\")"=w407) -> ("States Out"=w406:string)  [unwired: 14 in]
      }
      frame "SMO: Start Instrument UI" {
        # "Do not put any code in this frame.\n(It is a separator no-op. You can make a copy of this frame to create a new Macro frame)"
        n146 = Unbundle By Name(w411) -> ("Instrument UI"=w410:refnum<class "Instrument UI.lvclass">)
        n147 = call <vilib>:"Start.vi"("error in (no error)"=w409, "SMO"=w410) -> ("error out"=w408:errorcluster)  [unwired: 8 in, 1 out]
        n148 = call <vilib>:"Add State(s) to Queue__jki_lib_state_machine.vi"("State(s) in (\"\")"=w414) -> ("States Out"=w413:string)  [unwired: 14 in]
      }
      frame "SMO: Show Instrument UI" {
        # "Do not put any code in this frame.\n(It is a separator no-op. You can make a copy of this frame to create a new Macro frame)"
        n149 = Unbundle By Name(w422) -> ("Instrument UI"=w420:refnum<class "Instrument UI.lvclass">)
        n150 = call <vilib>:"GetState.vi"("error in (no error)"=w418, "SMO"=w420) -> ("error out"=w416:errorcluster, "SMO State"=w415:T1, "SMO out"=w419:refnum<class "Instrument UI.lvclass">)  [unwired: 7 in]
        n151 = call <vilib>:"Clear Errors.vi"("error in (no error)"=w416) -> ("error out"=w417:errorcluster)  [unwired: 5 in, 1 out]
        n152 = case shown="Default" w415 {
          tunnel: [w426 w429] -> w421
          tunnel: w419 -> [_ w428]
          tunnel: w417 -> [w426 w427]
          frame Default {
          }
          frame "Started" {
            n153 = call <vilib>:"Show.vi"("error in (no error)"=w427, "SMO.UI"=w428) -> ("error out"=w429:errorcluster)  [unwired: 8 in, 1 out]
          }
        }
        n154 = call <vilib>:"Add State(s) to Queue__jki_lib_state_machine.vi"("State(s) in (\"\")"=w425) -> ("States Out"=w424:string)  [unwired: 14 in]
      }
      frame "SMO: Destroy Instrument" {
        # "Do not put any code in this frame.\n(It is a separator no-op. You can make a copy of this frame to create a new Macro frame)"
        n155 = Unbundle By Name(w437) -> ("Instrument"=w435:refnum<class "Inst.Transport.lvclass">)
        n156 = call <vilib>:"GetState.vi"("error in (no error)"=w432, "SMO"=w435) -> ("error out"=w431:errorcluster, "SMO State"=w434:T1, "SMO out"=w430:refnum<class "Inst.Transport.lvclass">)  [unwired: 7 in]
        n157 = call <vilib>:"Clear Errors.vi"("error in (no error)"=w431) -> ("error out"=w433:errorcluster)  [unwired: 5 in, 1 out]
        n158 = case shown="\"Stopped\"" w434 {
          tunnel: [w441 w444] -> w436
          tunnel: w433 -> [w441 w443]
          tunnel: w430 -> [_ w442]
          frame Default {
          }
          frame "Stopped" {
            n159 = call <vilib>:"Destroy.vi"("error in (no error)"=w443, "SMO"=w442) -> ("error out"=w444:errorcluster)  [unwired: 9 in]
          }
        }
        n160 = call <vilib>:"Add State(s) to Queue__jki_lib_state_machine.vi"("State(s) in (\"\")"=w440) -> ("States Out"=w439:string)  [unwired: 14 in]
      }
      frame "SMO: Hide Instrument UI" {
        # "Do not put any code in this frame.\n(It is a separator no-op. You can make a copy of this frame to create a new Macro frame)"
        n161 = Unbundle By Name(w452) -> ("Instrument UI"=w450:refnum<class "Instrument UI.lvclass">)
        n162 = call <vilib>:"GetState.vi"("error in (no error)"=w448, "SMO"=w450) -> ("error out"=w446:errorcluster, "SMO State"=w445:T1, "SMO out"=w449:refnum<class "Instrument UI.lvclass">)  [unwired: 7 in]
        n163 = call <vilib>:"Clear Errors.vi"("error in (no error)"=w446) -> ("error out"=w447:errorcluster)  [unwired: 5 in, 1 out]
        n164 = case shown="\"Started\"" w445 {
          tunnel: [w456 w459] -> w451
          tunnel: w449 -> [_ w458]
          tunnel: w447 -> [w456 w457]
          frame Default {
          }
          frame "Started" {
            n165 = call <vilib>:"Hide.vi"("error in (no error)"=w457, "SMO.UI"=w458) -> ("error out"=w459:errorcluster)  [unwired: 8 in, 1 out]
          }
        }
        n166 = call <vilib>:"Add State(s) to Queue__jki_lib_state_machine.vi"("State(s) in (\"\")"=w455) -> ("States Out"=w454:string)  [unwired: 14 in]
      }
      frame "SMO: Stop Instrument UI" {
        # "Do not put any code in this frame.\n(It is a separator no-op. You can make a copy of this frame to create a new Macro frame)"
        n167 = Unbundle By Name(w466) -> ("Instrument UI"=w461:refnum<class "Instrument UI.lvclass">)
        n168 = call <vilib>:"GetState.vi"("error in (no error)"=w465, "SMO"=w461) -> ("error out"=w464:errorcluster, "SMO State"=w462:T1, "SMO out"=w460:refnum<class "Instrument UI.lvclass">)  [unwired: 7 in]
        n169 = call <vilib>:"Clear Errors.vi"("error in (no error)"=w464) -> ("error out"=w463:errorcluster)  [unwired: 5 in, 1 out]
        n170 = case shown="\"Created\", \"Started\"" w462 {
          tunnel: [w471 w474] -> w467
          tunnel: w460 -> [_ w473]
          tunnel: w463 -> [w471 w472]
          frame Default {
          }
          frame "Created", "Started" {
            n171 = call <vilib>:"Stop.vi"("error in (no error)"=w472, "SMO"=w473) -> ("error out"=w474:errorcluster)  [unwired: 8 in, 1 out]
          }
        }
        n172 = call <vilib>:"Add State(s) to Queue__jki_lib_state_machine.vi"("State(s) in (\"\")"=w470) -> ("States Out"=w469:string)  [unwired: 14 in]
      }
      frame "SMO: Stop Instrument" {
        # "Do not put any code in this frame.\n(It is a separator no-op. You can make a copy of this frame to create a new Macro frame)"
        n173 = Unbundle By Name(w483) -> ("Instrument"=w478:refnum<class "Inst.Transport.lvclass">)
        n174 = call <vilib>:"GetState.vi"("error in (no error)"=w482, "SMO"=w478) -> ("error out"=w481:errorcluster, "SMO State"=w479:T1, "SMO out"=w477:refnum<class "Inst.Transport.lvclass">)  [unwired: 7 in]
        n175 = call <vilib>:"Clear Errors.vi"("error in (no error)"=w481) -> ("error out"=w480:errorcluster)  [unwired: 5 in, 1 out]
        n176 = case shown="\"Created\", \"Started\"" w479 {
          tunnel: [w488 w491] -> w484
          tunnel: w477 -> [_ w490]
          tunnel: w480 -> [w488 w489]
          frame Default {
          }
          frame "Created", "Started" {
            n177 = call <vilib>:"Stop.vi"("error in (no error)"=w489, "SMO"=w490) -> ("error out"=w491:errorcluster)  [unwired: 8 in, 1 out]
          }
        }
        n178 = local write "UI"(FALSE ("UI")) -> ()
        n179 = property on="UI" class="Bool (strict)"("Visible"=FALSE) -> ()  [unwired: 2 in, 2 out]
        n180 = call <vilib>:"Add State(s) to Queue__jki_lib_state_machine.vi"("State(s) in (\"\")"=w487) -> ("States Out"=w486:string)  [unwired: 14 in]
      }
      frame "SMO: Destroy Instrument UI" {
        # "Do not put any code in this frame.\n(It is a separator no-op. You can make a copy of this frame to create a new Macro frame)"
        n181 = Unbundle By Name(w498) -> ("Instrument UI"=w497:refnum<class "Instrument UI.lvclass">)
        n182 = call <vilib>:"GetState.vi"("error in (no error)"=w495, "SMO"=w497) -> ("error out"=w494:errorcluster, "SMO State"=w492:T1, "SMO out"=w496:refnum<class "Instrument UI.lvclass">)  [unwired: 7 in]
        n183 = call <vilib>:"Clear Errors.vi"("error in (no error)"=w494) -> ("error out"=w493:errorcluster)  [unwired: 5 in, 1 out]
        n184 = case shown="\"Stopped\"" w492 {
          tunnel: w493 -> [w503 w506]
          tunnel: [w503 w505] -> w499
          tunnel: w496 -> [_ w504]
          frame Default {
          }
          frame "Stopped" {
            n185 = call <vilib>:"Destroy.vi"("error in (no error)"=w506, "SMO"=w504) -> ("error out"=w505:errorcluster)  [unwired: 9 in]
          }
        }
        n186 = call <vilib>:"Add State(s) to Queue__jki_lib_state_machine.vi"("State(s) in (\"\")"=w502) -> ("States Out"=w501:string)  [unwired: 14 in]
      }
      frame "---------- Splash ----------" {
        # "Template Separator\n(You can make a copy of, or modify, this frame)"
        n187 = call <vilib>:"Add State(s) to Queue__jki_lib_state_machine.vi"("State(s) in (\"\")"=w511) -> ("States Out"=w510:string)  [unwired: 14 in]
      }
      frame "Splash: Set Status" {
        # "Your code here.\n(You can make a copy of, or modify, this frame)"
        n188 = property on="Splash Status" class="Str"(error in=w514, "Value"=w515) -> (error out=w513:errorcluster)  [unwired: 1 in, 1 out]
        n189 = call <vilib>:"Add State(s) to Queue__jki_lib_state_machine.vi"("State(s) in (\"\")"=w518) -> ("States Out"=w517:string)  [unwired: 14 in]
      }
      frame "Splash: 2" {
        # "Your code here.\n(You can make a copy of, or modify, this frame)"
        n190 = call <vilib>:"Add State(s) to Queue__jki_lib_state_machine.vi"("State(s) in (\"\")"=w523) -> ("States Out"=w522:string)  [unwired: 14 in]
      }
    }
  }
  "error out" <- w2
